vi "Add Local Variable (Double).vi"(8 "error in (no error)":errorcluster, 9 "Value":dbl, 10 "Identifier":string, 11 "Sequence Ref in":refnum<k24>) -> (0 "error out":errorcluster, 3 "Sequence Ref out":refnum<k24>)   [LabVIEW 2015, in "Simple Sequence Tools - Editor.lvlib"]
uses:
  Simple Sequence Tools - Editor.lvlib
  NationalInstruments.VeriStand.RealTimeSequenceDefinitionApi
  NationalInstruments.VeriStand.DataTypes
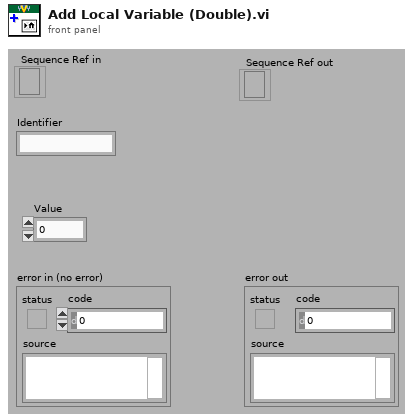
[diagram p1: front panel]
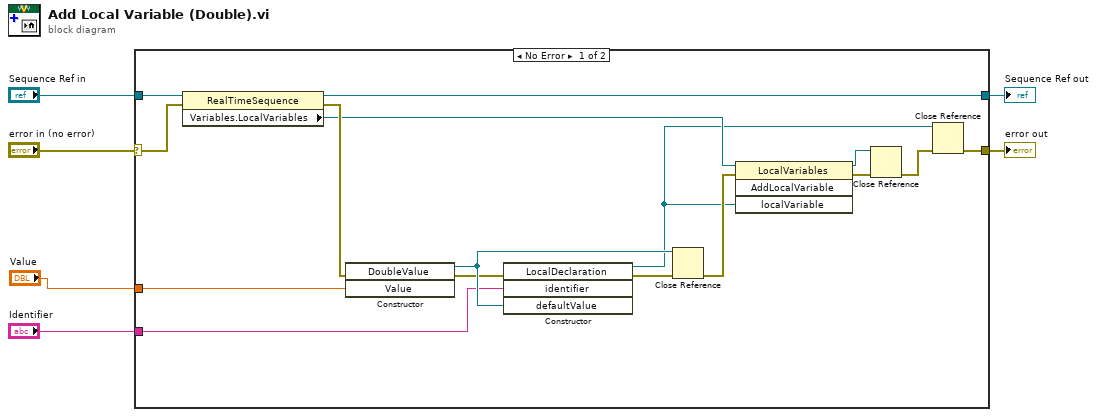
[diagram p0: block diagram]
diagram:
  n1 = case shown="No Error" "error in (no error)" {
    selector: "error in (no error)" -> [w8 w23]
    tunnel: "Identifier" -> [w17 _]
    tunnel: "Sequence Ref in" -> [w16 w24]
    tunnel: [w15 w24] -> w4
    tunnel: [w11 w23] -> w3
    tunnel: "Value" -> [w7 _]
    frame No Error {
      n2 = property class="RealTimeSequence"(reference=w16, error in=w8) -> (reference out=w15:refnum<k24>, error out=w19:errorcluster, "Variables.LocalVariables"=w18:refnum<k24>)
      n3 = constructor class="DoubleValue"(error in=w19, "Value"=w7) -> (reference out=w21:refnum<k24>, error out=w20:errorcluster)  [unwired: 2 in, 2 out]
      n4 = constructor class="LocalDeclaration"(error in=w20, "identifier"=w17, "defaultValue"=w21) -> (reference out=w9:refnum<k24>, error out=w14:errorcluster)  [unwired: 2 in, 3 out]
      n5 = Close Reference(reference=w21, error in (no error)=w14) -> (error out=w22:errorcluster)
      n6 = invoke class="LocalVariables" method="AddLocalVariable"(reference=w18, error in=w22, "localVariable"=w9) -> (reference out=w10:refnum<k24>, error out=w13:errorcluster)  [unwired: 1 in, 2 out]
      n7 = Close Reference(reference=w10, error in (no error)=w13) -> (error out=w12:errorcluster)
      n8 = Close Reference(reference=w9, error in (no error)=w12) -> (error out=w11:errorcluster)
    }
    frame Error {
    }
  }
  "Sequence Ref out" <- w4
  "error out" <- w3
